vi "CAN Frames Write.vi"(7 "Channel Number":u32, 8 "error in (no error)":errorcluster, 9 "Timeout (ms)":i32=1000, 10 "Frames":T2[](array[typedef]) {"payload" format="%x"; "timestamp" format="%<%.7X\n%x>T"; "type" items=["CAN Data"=0, "CAN Remote"=1, "CAN Bus Error"=2, "CAN 2.0 Data"=8, "CAN FD Data"=16, "CAN FD+BRS Data"=24, "J1939 Data"=192, "Delay"=224, "Log Trigger"=225, "Start Trigger"=226]; "identifier" format="%x"}, 11 "FPGA Refnum":T1) -> (0 "error out":errorcluster)   [LabVIEW 2020, in "985x Support Addon Engine.lvlib"]
uses:
  985x Support Addon Engine.lvlib
  <vilib>/xnet/xnet.llb/XNET Frame CAN.ctl
  <vilib>/xnet/xnet.llb/XNET Frame Type CAN.ctl
  Types/FPGA Refnum.ctl
  <vilib>/Utility/error.llb/Error Cluster From Error Code.vi
  <vilib>/rvi/errors/niLvFpgaAdjustHostInterfaceError.vi
  <vilib>/rvi/interface/nirviMethod/nirviMethod.xnode
  <vilib>/FPGAPlugInAG/Dynamic/niLvFpga_WriteFifo_Dynamic.vi
  <vilib>/rvi/errors/niLvFpgaMergeErrorWithErrorCode.vi
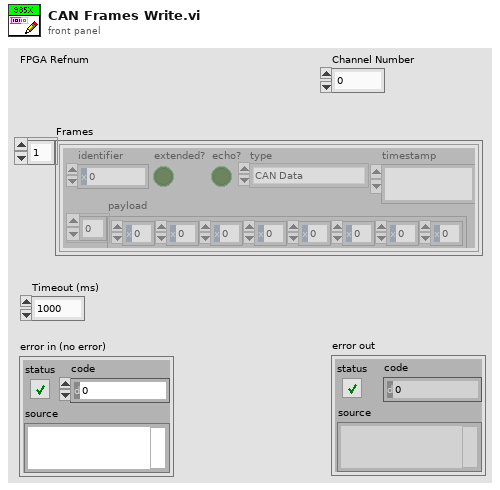
[diagram p1: front panel]
types:
  T1 = typedef "985x Support Addon Engine.lvlib/FPGA Refnum.ctl" = refnum<k20>
  T2 = typedef "XNET Frame CAN.ctl" = cluster{"timestamp":timestamp, "payload":u8[], "identifier":u32, "type":T3, "extended?":bool, "echo?":bool}
  T3 = typedef "XNET Frame Type CAN.ctl" = u8
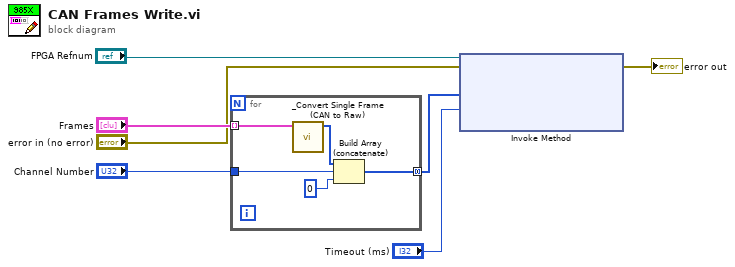
[diagram p0: block diagram]
diagram:
  n1 = for {
    tunnel: "Frames" -> [w12] mode=indexing
    tunnel: "Channel Number" -> [w9]
    tunnel: [w8] -> w2 mode=concatenating
    n2 = call "_Convert Single Frame (CAN to Raw).vi"("CAN frame"=w12) -> ("Raw U32"=w10:u32[])  [unwired: 9 in, 1 out]
    n3 = Build Array (concatenate)(w10, w9, u32 0) -> (w8:u32[])
  }
  n4 = xnode "Invoke Method"("FPGA VI Reference In"="FPGA Refnum", "error in"="error in (no error)", "Data"=w2, "Timeout (ms)"="Timeout (ms)") -> ("error out"=→"error out":errorcluster)  [unwired: 2 out]
